vi "FluxCreate.vi"(2 "Endereço slave":u16=1, 3 "Recurso VISA":refnum<visa-resource-name>) -> (0 "Error Out":errorcluster, 1 "Master Out":refnum<class "Modbus Master.lvclass">)   [LabVIEW 2019]
uses:
  <vilib>/Modbus/master/Modbus Master.lvclass
  <vilib>/Modbus/master/Create Master Instance (Serial).vi
panel:
  # "Entrada"
  # "Saída"
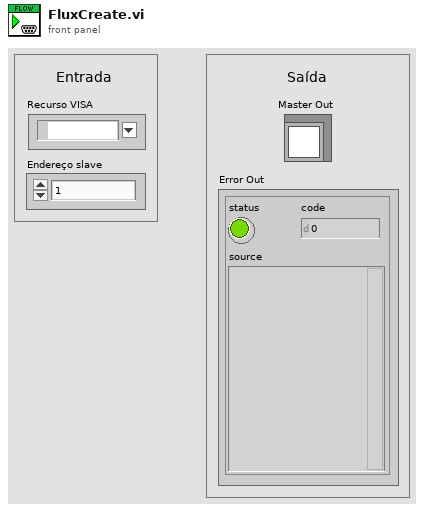
[diagram p1: front panel]
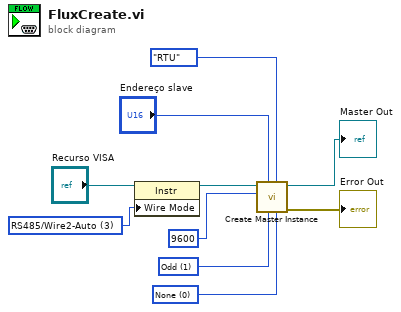
[diagram p0: block diagram]
diagram:
  w9 = i16 3 items=["Unknown"=-1, "RS485/Wire4"=0, "RS485/Wire2-EchoDTR"=1, "RS485/Wire2-CtrlDTR"=2, "RS485/Wire2-Auto"=3, "RS232/DTE"=128, "RS232/DCE"=129, "RS232/AUTO"=130] ("Serial Settings:Wire Mode")
  w5 = u16 0 items=["None", "XON/XOFF", "RTS/CTS", "XON/XOFF & RTS/CTS", "DTR/DSR", "XON/XOFF & DTR/DSR"] ("Flow Control")
  w6 = u16 1 items=["None", "Odd", "Even", "Mark", "Space"] ("Parity")
  n1 = property class="Instr"(reference="Recurso VISA", "Wire Mode"=w9) -> (reference out=w8:refnum<visa-resource-name>)  [unwired: 1 in, 1 out]
  n2 = call-poly <vilib>:"Create Master Instance.vi"("flow control (None)"=w5, "serial type"=enum16{"RTU", "ASCII"}."RTU" ("Mode"), "parity (Even)"=w6, "unit ID"="Endereço slave", "baud rate (9600)"=u32 9600 ("Baud Rate"), "VISA resource name"=w8) -> ("error out"=→"Error Out":errorcluster, "serial master instance"=→"Master Out":refnum<class "Modbus Master.lvclass">)  [unwired: 4 in]
